vi "File Read Orbit.vi"(8 "error in (no error)":errorcluster, 11 "file path (dialog if empty)":path) -> (0 "error out":errorcluster, 2 "BPM Reading Names":string[](array[string]), 3 "Orbit":dbl[](array[numeric]))   [LabVIEW 2011, in "File VIs.lvlib"]
doc: "Reads an \"Orbit\" text file and converts the data to a 1D, double-precision array of numbers.\n\nFile format:\nColumn 1: BPM names\nColumn 2: Position value (mm)\nColumn separator: <TAB> character\n\nEx.:\nAMP01BH<TAB>2.28541931\nAMP02AH<TAB>-0.05323151\nAMP01BV<TAB>-4.67227631\nAMP02AV<TAB>-4.66651489"
uses:
  File VIs.lvlib
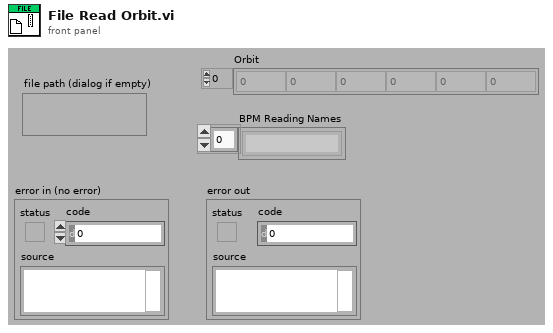
[diagram p1: front panel]
types:
  T1 = enum16{"open", "replace", "create", "open or create", "replace or create", "replace or create with confirmation"}
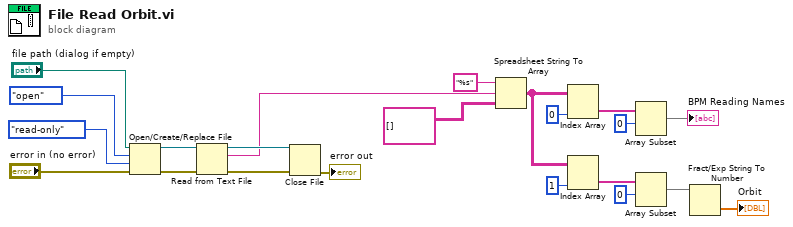
[diagram p0: block diagram]
diagram:
  n1 = Open/Create/Replace File(file path (use dialog)="file path (dialog if empty)", error in="error in (no error)", operation (0:open)=T1."open", access (0:read/write)=enum16{"read/write", "read-only", "write-only"}."read-only") -> (refnum out=w17:refnum<file>, error out=w16:errorcluster)  [unwired: 2 in, 1 out]
  n2 = Read from Text File(file (use dialog)=w17, error in=w16) -> (refnum out=w15:refnum<file>, text=w11:string, error out=w14:errorcluster)  [unwired: 2 in, 1 out]
  n3 = Close File(refnum=w15, error in=w14) -> (error out=→"error out":errorcluster)  [unwired: 1 out]
  n4 = Spreadsheet String To Array(format string="%s", spreadsheet string=w11, array type (2D Dbl)=string[][] []) -> (array=w3:string[][])  [unwired: 1 in]
  n5 = Index Array(array=w3, index (col)=0 ("index (row)")) -> (element=w9:string[])  [unwired: 1 in]
  n6 = Index Array(array=w3, index (col)=1 ("index (row)")) -> (element=w5:string[])  [unwired: 1 in]
  n7 = Array Subset(array=w9, index=0) -> (→"BPM Reading Names":string[])  [unwired: 1 in]
  n8 = Array Subset(array=w5, index=0) -> (w2:string[])  [unwired: 1 in]
  n9 = Fract/Exp String To Number(string=w2) -> (number=→"Orbit":dbl[])  [unwired: 3 in, 1 out]
